vi "WPILogGetHeaderInfo.vi"(8 "error in (no error)":errorcluster, 11 "Data Value Reference in":refnum<data-value>) -> (0 "error out":errorcluster, 1 "Header Extra String":string, 2 "Version":dbl, 3 "Boolean":bool)   [LabVIEW 2020]
uses:
  Typedef/WPILibLog.ctl
  Typedef/Header.ctl
  Typedef/Entry.ctl
  Typedef/Record.ctl
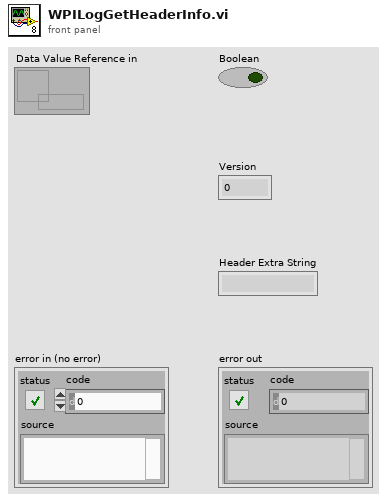
[diagram p1: front panel]
types:
  T1 = typedef "WPILibLog.ctl" = cluster{"Header":T2, "Record Start Idx":i32, "Entries":map{u32, T3}, "file ref":refnum<file>, "Finished Entries":T3[], "raw data":u8[]}
  T2 = typedef "Header.ctl" = cluster{"Header String":string, "Version":dbl, "Header Extra String Length":u32, "Header Extra String":string}
  T3 = typedef "Entry.ctl" = cluster{"ID":u32, "Records":T4[], "Finished?":bool, "Name":string, "Type":string, "Metadata":string, "RecordCnt":i32}
  T4 = typedef "Record.ctl" = cluster{"raw data":u8[], "ID":u32, "Size (bytes)":u32, "Timestamp":u64}
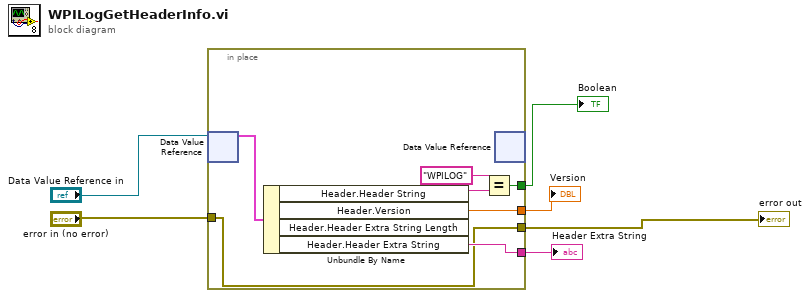
[diagram p0: block diagram]
diagram:
  n1 = in-place {
    in-place-border: [w12] -> w2
    in-place-border: [w11] -> w3
    in-place-border: [w8] -> w4
    in-place-border: "error in (no error)" -> [w7]
    in-place-border: [w7] -> w6
    n2 = in-place-dvr #1("Data Value Reference in") -> (w13:T1)  [unwired: 1 out]
    n3 = Unbundle By Name(w13) -> ("Header.Header String"=w10:string, "Header.Version"=w11:dbl, "Header.Header Extra String"=w12:string)  [unwired: 1 out]
    n4 = Equal?(x="WPILOG", y=w10) -> (x = y?=w8:bool)
    n5 = in-place-dvr #1() -> ()  [unwired: 1 in, 2 out]
  }
  "error out" <- w6
  "Boolean" <- w4
  "Version" <- w3
  "Header Extra String" <- w2
